vi "FGV-GlobalEventRef(lvlibp).vi"(6 "Operation":enum16{"Create", "Read", "Destroy"}(ring), 8 "error in (no error)":errorcluster, 9 "Timeout In ms (5000 ms)":i32, 10 "Force Destroy?":bool) -> (0 "error out":errorcluster, 3 "Event":refnum<user-event>)   [LabVIEW 2017, in "Communicable State Machine.lvlib"]
uses:
  Communicable State Machine.lvlib
  Typedef/_CSM_GlobalLog_MSG.ctl
  Typedef/_CSM_Response Source Message.ctl
  Typedef/_CSM_GlobalLog_MSG_TYPE.ctl
  FGV-GlobalEventRef.vi
  _Shared/CSM Shared.lvlib
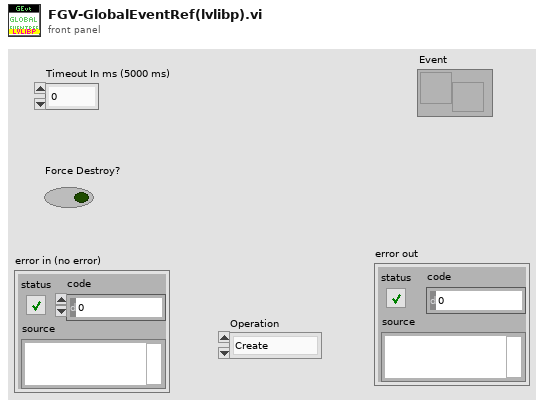
[diagram p1: front panel]
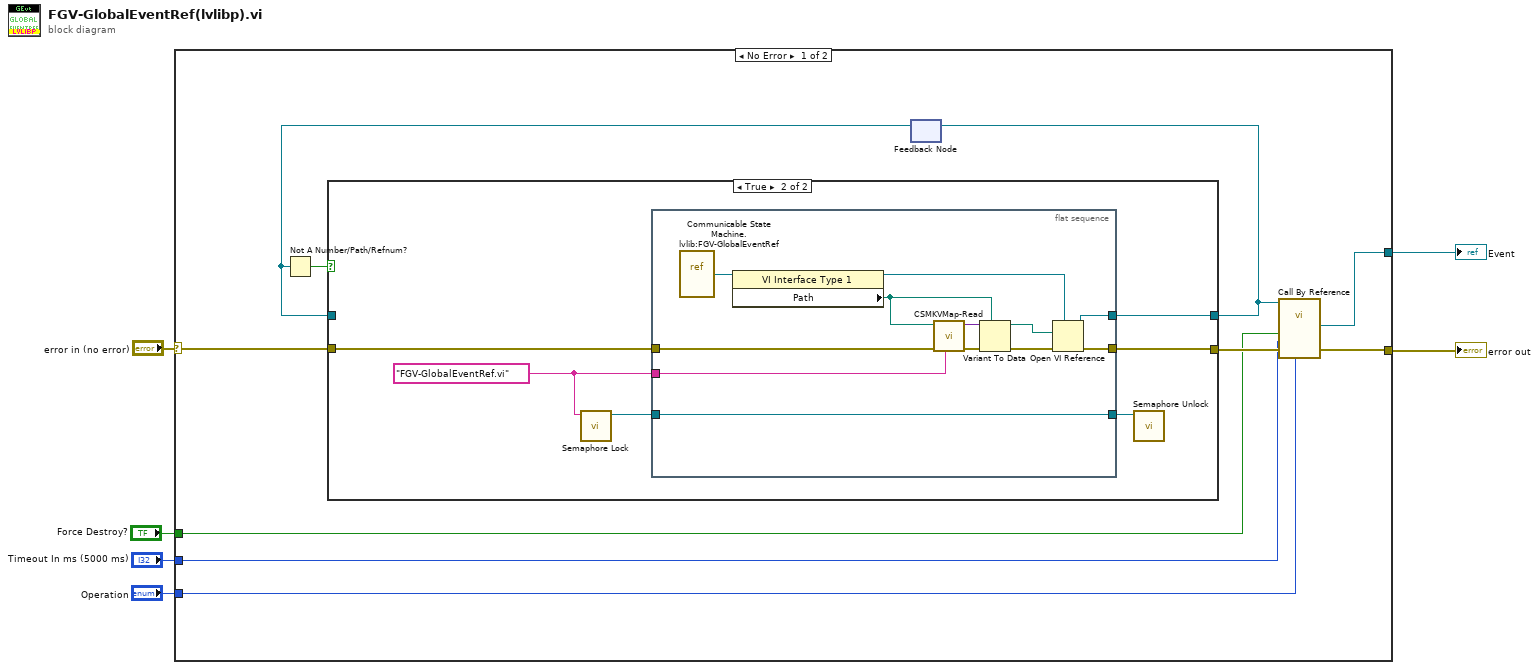
[diagram p0: block diagram]
diagram:
  n1 = case shown="No Error" "error in (no error)" {
    selector: "error in (no error)" -> [w12 w37]
    tunnel: [w10 _] -> w6
    tunnel: [w11 w37] -> w4
    tunnel: "Operation" -> [w7 _]
    tunnel: "Timeout In ms (5000 ms)" -> [w9 _]
    tunnel: "Force Destroy?" -> [w8 _]
    frame No Error {
      n2 = feedback #1() -> (w15:refnum<vi>)  [unwired: 1 in]
      n3 = Not A Number/Path/Refnum?(number/path/refnum=w15) -> (NaN/Path/Refnum?=w16:bool)
      n4 = case shown="True" w16 {
        tunnel: [w17 w23] -> w14
        tunnel: [w18 w24] -> w13
        tunnel: w12 -> [w18 w22]
        tunnel: w15 -> [w17 _]
        frame False {
        }
        frame True {
          w19 = "FGV-GlobalEventRef.vi" ("name")
          n5 = call "Semaphore Lock.vi"("name"=w19) -> ("semaphore"=w20:refnum<queue>)  [unwired: 10 in]
          n6 = flat-sequence {
            tunnel: [w32] -> w24
            tunnel: [w30] -> w23
            tunnel: w22 -> [w28]
            tunnel: [w26] -> w21
            tunnel: w20 -> [w26]
            tunnel: w19 -> [w25]
            frame #0 {
              n7 = vi-ref "Communicable State Machine.lvlib:FGV-GlobalEventRef.vi"() -> (w27:refnum<vi>)
              n8 = property class="VI Interface Type 1"(reference=w27) -> (reference out=w29:refnum<vi>, "Path"=w31:path)  [unwired: 1 in, 1 out]
              n9 = call "CSMKVMap-Read.vi"("name"=w25, "Error in"=w28, "default value (empty variant)"=w31) -> ("Error out"=w36:errorcluster, "value"=w35:variant)  [unwired: 5 in]
              n10 = Variant To Data(error in=w36, type=w31, Variant=w35) -> (data=w34:path, error out=w33:errorcluster)
              n11 = Open VI Reference(type specifier VI Refnum (for type only)=w29, vi path=w34, error in (no error)=w33) -> (vi reference=w30:refnum<vi>, error out=w32:errorcluster)  [unwired: 3 in]
            }
          }
          n12 = call "Semaphore Unlock.vi"("semaphore"=w21) -> ()  [unwired: 11 in]
        }
      }
      n13 = feedback-in #1(w14) -> ()
      n14 = call-by-ref "?"(reference=w14, "Operation"=w7, "error in (no error)"=w13, "Timeout In ms (5000 ms)"=w9, "Force Destroy?"=w8) -> ("error out"=w11:errorcluster, "Event"=w10:refnum<user-event>)  [unwired: 7 in, 2 out]
    }
    frame Error {
    }
  }
  "Event" <- w6
  "error out" <- w4
